vi "OnMLine.vi"(11 "Start Goal Data":T1) -> (1 "On the Line?":bool, 2 "Match Index":i32, 3 "Start Goal Data out":T1)   [LabVIEW 2013]
uses:
  Bug_StartGoalData.ctl
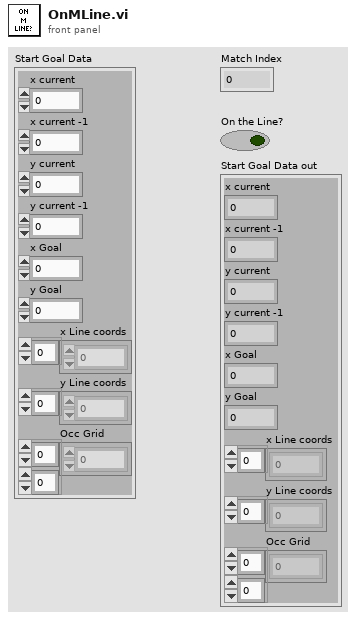
[diagram p1: front panel]
types:
  T1 = typedef "Bug_StartGoalData.ctl" = cluster{"x current":i32, "x current -1":i32, "y current":i32, "y current -1":i32, "x Goal":i32, "y Goal":i32, "x Line coords":i32[], "y Line coords":i32[], "Occ Grid":dbl[][]}
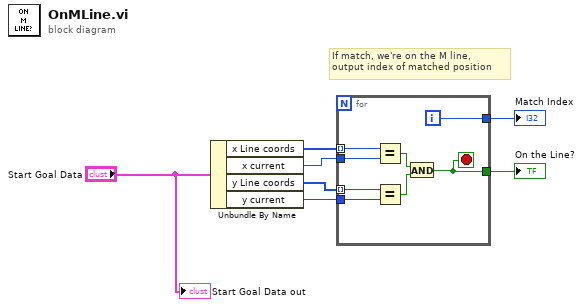
[diagram p0: block diagram]
diagram:
  # "If match, we're on the M line,\noutput index of matched position"
  n1 = Unbundle By Name("Start Goal Data") -> ("x Line coords"=w5:i32[], "x current"=w3:i32, "y Line coords"=w4:i32[], "y current"=w2:i32)
  n2 = for {
    tunnel: w5 -> [w15] mode=indexing
    tunnel: w4 -> [w14] mode=indexing
    tunnel: w3 -> [w13]
    tunnel: w2 -> [w12]
    tunnel: [w8] -> w6
    tunnel: [w11] -> w7
    i -> [w11]
    stop <- w8 stop-if-true
    n3 = Equal?(x=w15, y=w13) -> (x = y?=w10:bool)
    n4 = Equal?(x=w14, y=w12) -> (x = y?=w9:bool)
    n5 = And(x=w10, y=w9) -> (x .and. y?=w8:bool)
  }
  "Match Index" <- w7
  "On the Line?" <- w6
  "Start Goal Data out" <- "Start Goal Data"
